vi "Get RPC Type Descriptor.vi"(8 "error in (no error)":errorcluster, 10 "Function Block#Method":string, 11 "TwinCAT ADS in":refnum<class "TwinCAT ADS.lvclass">) -> (0 "error out":errorcluster, 2 "RPC Type Descriptor":T1, 3 "TwinCAT ADS out":refnum<class "TwinCAT ADS.lvclass">)   [LabVIEW 2018, in "TwinCAT ADS.lvclass"]
uses:
  TwinCAT ADS.lvclass
  Controls/PLC RPC Type Descriptor.ctl
  Controls/PLC RPC Parameter Type Descriptor.ctl
  TwinCAT ADS.lvclass/TwinCAT ADS.ctl
  TwinCAT.Ads
  Get From Symbol Map.vi
  Get From Symbol Map Daemon.vi
  Get Symbol Map.vi
  Format String.vi
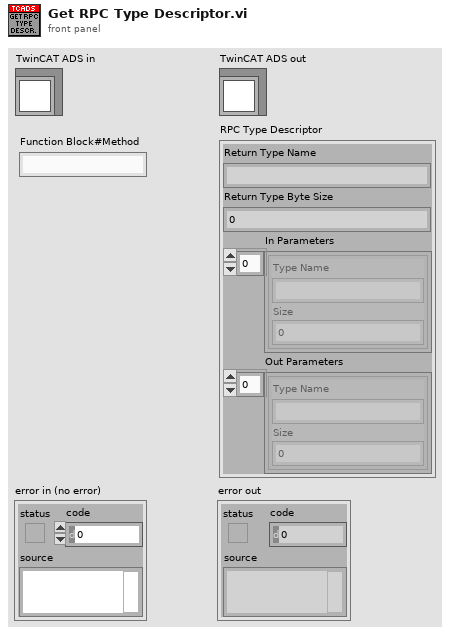
[diagram p1: front panel]
types:
  T1 = typedef "TwinCAT ADS.lvclass/PLC RPC Type Descriptor.ctl" = cluster{"Return Type Name":string, "Return Type Byte Size":i32, "In Parameters":T2[], "Out Parameters":T2[]}
  T2 = typedef "TwinCAT ADS.lvclass/PLC RPC Parameter Type Descriptor.ctl" = cluster{"Type Name":string, "Size":i32}
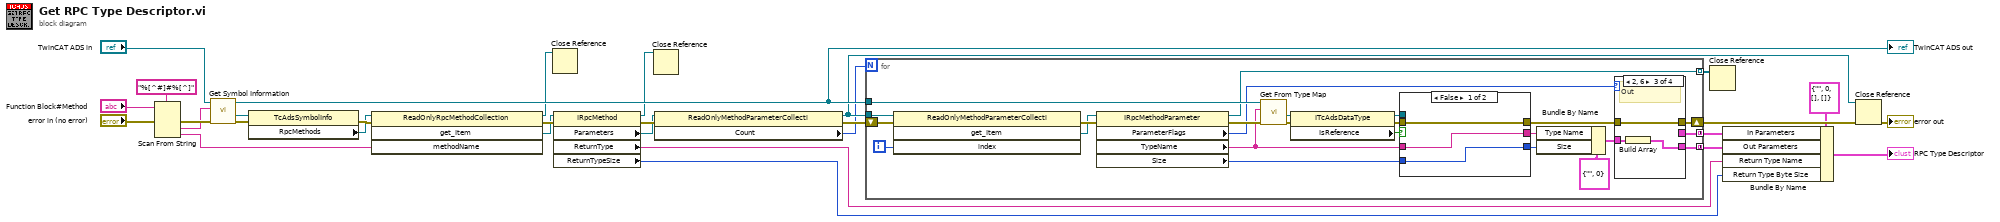
[diagram p0: block diagram]
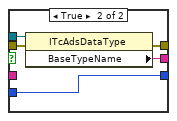
[diagram p2: hidden frame]
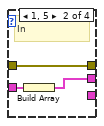
[diagram p4: hidden frame]
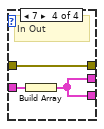
[diagram p5: hidden frame]
diagram:
  n1 = Scan From String(format string="%[^#]#%[^]" ("regular expression"), input string="Function Block#Method", error in="error in (no error)") -> (error out=w5:errorcluster, output 1=w2:string, output 2=w18:string)  [unwired: 3 in, 2 out]
  n2 = call "Get Symbol Information.vi"("error in (no error)"=w5, "Symbol Name"=w2, "TwinCAT ADS in"="TwinCAT ADS in") -> ("error out"=w6:errorcluster, ".NET Symbol Information"=w3:refnum<k24>, "TwinCAT ADS out"=w29:refnum<class "TwinCAT ADS.lvclass">)  [unwired: 6 in]
  "TwinCAT ADS out" <- w29
  n3 = property class="TcAdsSymbolInfo"(reference=w3, error in=w6) -> (error out=w19:errorcluster, "RpcMethods"=w17:refnum<k24>)  [unwired: 1 out]
  n4 = invoke class="ReadOnlyRpcMethodCollection" method="get_Item"(reference=w17, error in=w19, "methodName"=w18) -> (reference out=w11:refnum<k24>, error out=w13:errorcluster, "get_Item"=w12:refnum<k24>)  [unwired: 1 in, 1 out]
  n5 = Close Reference(reference=w11) -> ()  [unwired: 1 in, 1 out]
  n6 = property class="IRpcMethod"(reference=w12, error in=w13) -> (reference out=w7:refnum<k24>, error out=w27:errorcluster, "Parameters"=w26:refnum<k24>, "ReturnType"=w9:string, "ReturnTypeSize"=w8:i32)
  n7 = Close Reference(reference=w7) -> ()  [unwired: 1 in, 1 out]
  n8 = property class="ReadOnlyMethodParameterCollecti"(reference=w26, error in=w27) -> (reference out=w20:refnum<k24>, error out=w22:errorcluster, "Count"=w1:i32)
  n9 = for {
    N: w1 -> [_]
    shift-right: [w42] -> w30
    shift-left: w22 -> [w51]
    tunnel: [w44] -> w24 mode=concatenating
    tunnel: w20 -> [w48]
    tunnel: [w46] -> w21 mode=indexing
    tunnel: [w43] -> w10 mode=concatenating
    tunnel: w29 -> [w53]
    i -> [w50]
    n10 = invoke class="ReadOnlyMethodParameterCollecti" method="get_Item"(reference=w48, error in=w51, "index"=w50) -> (error out=w49:errorcluster, "get_Item"=w47:refnum<k24>)  [unwired: 1 in, 2 out]
    n11 = property class="IRpcMethodParameter"(reference=w47, error in=w49) -> (reference out=w46:refnum<k24>, error out=w52:errorcluster, "ParameterFlags"=w45:u32, "TypeName"=w34:string, "Size"=w33:i32)
    n12 = call "Get From Type Map.vi"("error in (no error)"=w52, "Type Name"=w34, "TwinCAT ADS in"=w53) -> ("error out"=w36:errorcluster, ".NET AdsDataType"=w37:refnum<k24>)  [unwired: 6 in, 1 out]
    n13 = property class="ITcAdsDataType"(reference=w37, error in=w36) -> (reference out=w40:refnum<k24>, error out=w39:errorcluster, "IsReference"=w38:bool)
    n14 = case shown="False" w38 {
      tunnel: w39 -> [w57 w62]
      tunnel: w40 -> [_ w61]
      tunnel: [w56 w60] -> w41
      tunnel: w34 -> [w56 _]
      tunnel: w33 -> [w55 w59]
      tunnel: [w57 w58] -> w54
      tunnel: [w55 w59] -> w32
      frame False {
      }
      frame True {
        n15 = property class="ITcAdsDataType"(reference=w61, error in=w62) -> (error out=w58:errorcluster, "BaseTypeName"=w60:string)  [unwired: 1 out]
      }
    }
    n16 = Bundle By Name(cluster=T2 {"Type Name"="", "Size"=0} ("Parameter"), "Type Name"=w41, "Size"=w32) -> (w31:T2)
    n17 = case shown="2, 6" w45 {
      tunnel: [_ w64 _ w70] -> w44
      tunnel: [_ _ w67 w70] -> w43
      tunnel: w54 -> [w63 w66 w69 w72]
      tunnel: w31 -> [_ w65 w68 w71]
      tunnel: [w63 w66 w69 w72] -> w42
      frame Default {
      }
      frame 1, 5 {
        # "In"
        n18 = Build Array(w65) -> (w64:T2[])
      }
      frame 2, 6 {
        # "Out"
        n19 = Build Array(w68) -> (w67:T2[])
      }
      frame 7 {
        # "In Out"
        n20 = Build Array(w71) -> (w70:T2[])
      }
    }
  }
  n21 = Close Reference(reference=w21) -> ()  [unwired: 1 in, 1 out]
  n22 = Bundle By Name(cluster=T1 {"Return Type Name"="", "Return Type Byte Size"=0, "In Parameters"=[], "Out Parameters"=[]} ("RPC Type Descriptor"), "In Parameters"=w24, "Out Parameters"=w10, "Return Type Name"=w9, "Return Type Byte Size"=w8) -> (→"RPC Type Descriptor":T1)
  n23 = Close Reference(reference=w20, error in (no error)=w30) -> (error out=→"error out":errorcluster)
